vi "校准数据文件路径.vi"() -> (3 "appended path":path)   [LabVIEW 2016, in "斯坦道总氮.lvlib"]
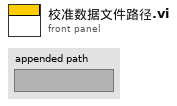
[diagram p1: front panel]
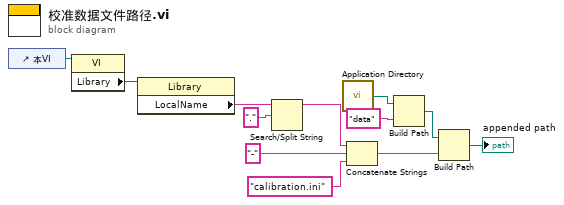
[diagram p0: block diagram]
diagram:
  n1 = control-ref of="本VI"() -> (w1:refnum<vi>)
  n2 = property class="VI"(reference=w1) -> ("Library"=w6:refnum<vi>)  [unwired: 1 in, 2 out]
  n3 = property class="Library"(reference=w6) -> ("LocalName"=w7:string)  [unwired: 1 in, 2 out]
  n4 = Search/Split String(string=w7, search string/char (-)="." ("搜索字符串/字符(-)")) -> (substring before match=w9:string)  [unwired: 1 in, 2 out]
  n5 = call <vilib>:"Application Directory.vi"() -> ("Application Directory"=w3:path)
  n6 = Concatenate Strings(w9, "-" ("字符串"), "calibration.ini" ("名称或相对路径")) -> (w12:string)
  n7 = Build Path(base path=w3, name or relative path="data" ("名称或相对路径")) -> (appended path=w4:path)
  n8 = Build Path(base path=w4, name or relative path=w12) -> (appended path=→"appended path":path)
